vi "Cache.Delete.vi"(7 "Idx":i32, 8 "error in":errorcluster, 10 "Files":path[](array[path]), 11 "Data in":T1) -> (0 "error out":errorcluster, 3 "Data out":T1)   [LabVIEW 2016]
doc: "Write test results (measurement values) to proda database\n\nWabco 2017 All right reserved\nAuthor: maciej.szupienko@wabco-auto.com"
uses:
  Cache.Data.ctl
  Cache.Data.Status.ctl
  Cache.Data.Sets.ctl
  Tools/EventLog/EventLog.EventSource.ctl
  Tools/Translator/Translator.Message.ctl
  Tools/EventLog/EventLog.New(single).vi
  Global/ApplicationGlobal.vi
  Tools/EventLog/EventLog.Buffer.vi
  Tools/EventLog/EventLog.File.ReadWrite.vi
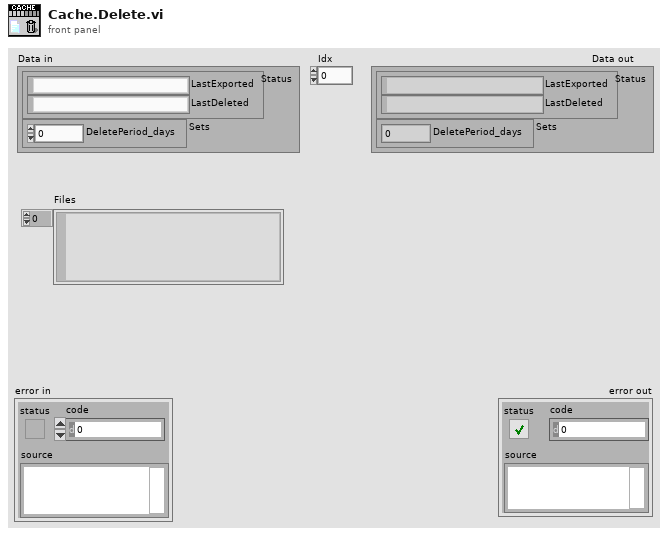
[diagram p1: front panel]
types:
  T1 = typedef "Cache.Data.ctl" = cluster{"Status":T2, "Sets":T3}
  T2 = typedef "Cache.Data.Status.ctl" = cluster{"LastExported":string, "LastDeleted":string}
  T3 = typedef "Cache.Data.Sets.ctl" = cluster{"DeletePeriod_days":dbl}
  T4 = typedef "Translator.Message.ctl" = enum16{"-", "Event confirmed", "Log out", "Log in", "Shutdown", "Cancel", "Start", "Continue", "Stop", "On", "Off", "OK", "NOK", "NOK %s", "This", "Prev", "Home", "Work", "In progress...", "Missing", "Empty", "Hardware failure", "Initial", "Error %d >> %s", "Error %d >> %s >> %s", "Starting %s", "Quitting %s", "Configured", "Initializing", "Quitting", "Loading", "Running %s", "Stopped", "Summary", "Do you want to continue?", "Do you want to exit?", "Log out?", "System", "All", "IDLE", "Translating...%s", "Not found", "Alarm %s", "Run", "Skip", "Abort", "Repeat", "Please wait...", "Database disconnected", "Login to database successful", "Login to database failed: %d; %s", "Get process step data for %s", "Changeover off", "Changeover into %s", "Product %s | %s found in cache with status %d at previous station", "Product %s | %s found in database with status %d at previous station", "Product %s | %s not found in cache at previous station", "Product %s | %s not found in database at previous station", "Product %s | %s found in cache with status %d at this station (%d repetion)", "Product %s | %s found in database with status %d at this station (%d repetition)", "Product %s | %s not found in cache at this station", "Product %s | %s not found in database at this station", "Product %s | %s found in cache for component %s | %s", "Product %s | %s found in database for component %s | %s", "Product not found in cache for component %s | %s", "Product not found in database for component %s | %s", "Product %s | %s connected with component %s | %s (cache)", "Product %s | %s connected with component %s | %s (database)", "New data for %s | %s (cache)", "New data for %s | %s (database)", "File %s moved (cache)", "File %s deleted (cache)", "Msg %d >> %s", "PLC LifeBit Failure", "Reconnecting DB", "Reconnecting PLC", "Free disk space is below 1GB - contact technician"}
  T5 = typedef "EventLog.EventSource.ctl" = enum16{"All", "Gui", "Cache", "PLC1", "PLC2", "PLC3", "DB", "DB01", "DB02", "DB03", "DB04", "DB05", "DB06", "DB07", "DB08", "DB09", "DB10", "DB11", "DB12", "DB13", "DB14", "DB15", "DB16"}
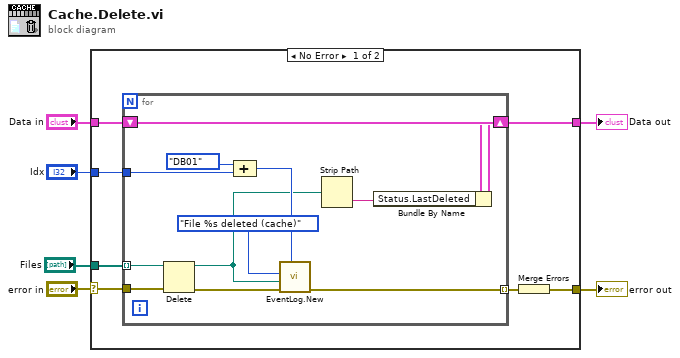
[diagram p0: block diagram]
diagram:
  n1 = case shown="No Error" "error in" {
    selector: "error in" -> [w12 w26]
    tunnel: [w9 w26] -> w6
    tunnel: "Idx" -> [w8 _]
    tunnel: "Files" -> [w11 _]
    tunnel: "Data in" -> [w7 w25]
    tunnel: [w7 w25] -> w1
    frame No Error {
      n2 = for {
        tunnel: w11 -> [w24] mode=indexing
        tunnel: w12 -> [w22]
        tunnel: [w23] -> w10 mode=indexing
        tunnel: w8 -> [w21]
        shift-right: [w13] -> _
        shift-left: w7 -> [w15]
        n3 = Delete(path (use dialog)=w24, error in=w22) -> (deleted path=w16:path, error out=w17:errorcluster)  [unwired: 3 in, 1 out]
        n4 = Compound Arithmetic op=unknown(EventLog.EventSource."DB01" ("Source (All)"), w21) -> (w18:i32)
        n5 = call-poly "EventLog.New.vi"("Source (All)"=w18, "error in (no error)"=w17, "Arg"=w16, "Message (-)"=Translator.Message."File %s deleted (cache)") -> ("error out"=w23:errorcluster)  [unwired: 6 in, 1 out]
        n6 = Strip Path(path=w16) -> (name=w14:string)  [unwired: 1 out]
        n7 = Bundle By Name(cluster=w15, "Status.LastDeleted"=w14) -> (w13:T1)
      }
      n8 = Merge Errors(w10) -> (w9:errorcluster)
    }
    frame Error {
    }
  }
  "error out" <- w6
  "Data out" <- w1
